vi "CalibrationOAM.vi"() -> ()   [LabVIEW 2015]
uses:
  <vilib>/Utility/file.llb/Write Delimited Spreadsheet (DBL).vi
panel:
  in  "Dimensions":i32=21
  in  "Steps":enum32{"One Step", "Two Step"}(radio)
  out "SLM  B":picture
  out "SLM A":picture
  out "Calibration Curve":dbl[](array[numeric])=[1.04866638e-09, 2.36400149e-10, 3.28397032e-10, 3.4456285e-11, 1.42615789e-11, 6.36260558e-11, 1.65061454e-11, 1.20186092e-11, 3.22117194e-11, 4.34313557e-11, 1.69085523e-10, -3.68856204e-12, 5.28650778e-12, -1.44559289e-12, 7.52947704e-12, 3.04194213e-12, 9.77404269e-12, 3.04194213e-12, 7.52947704e-12, 7.98972867e-13, 3.04194213e-12]
  out "Measured Power":dbl=1.53557755e-09
  out "Generated OAM Progress":u8(slide)=100 scale=0.0..100.0
  out "Current Measured OAM":i32=10
  in  "Measured OAM":i32[](array[numeric])=[-10, -9, -8, -7, -6, -5, -4, -3, -2, -1, 0, 1, 2, 3, 4, 5, 6, 7, 8, 9, 10]
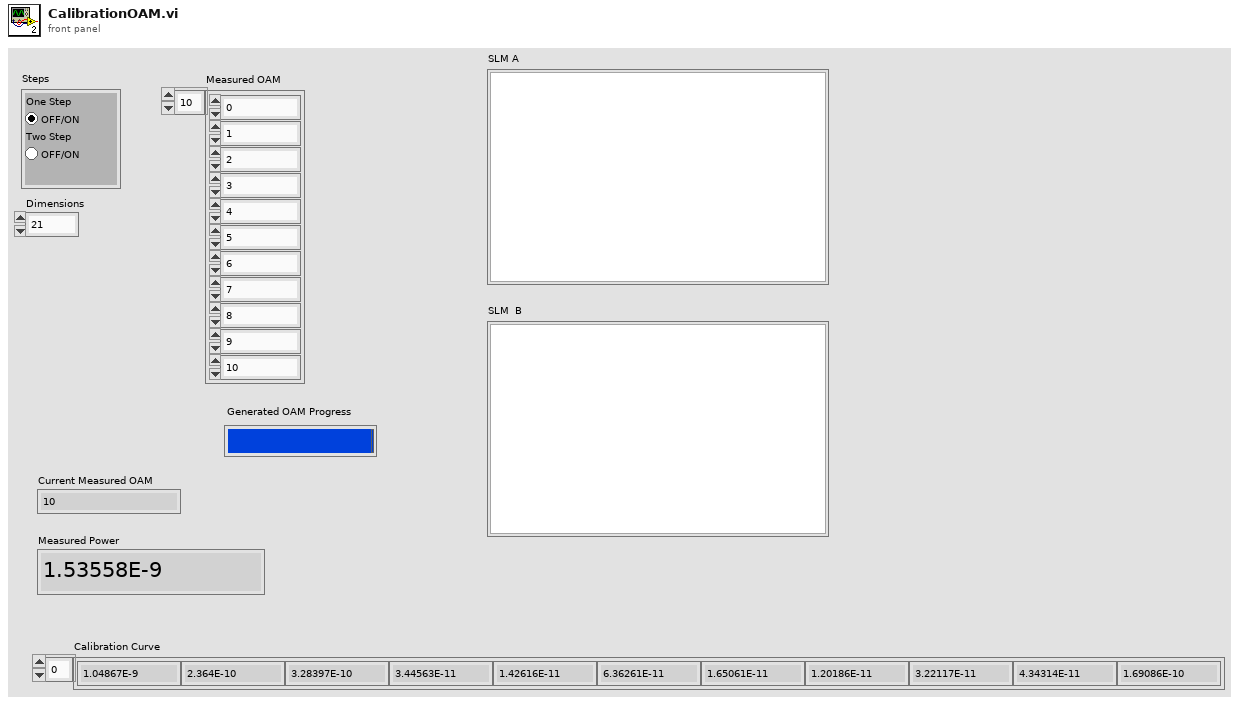
[diagram p1: front panel]
types:
  T1 = cluster{"type":enum16{"Azimuth Mode", "LG mode", "HG mode"}, i32, i32, dbl, dbl}
  T2 = cluster{"type":enum16{"Azimuth Mode", "LG mode", "HG mode"}, "Numeric":i32, i32, dbl, dbl}
  T3 = cluster{"type":enum16{"Azimuth Mode", "LG mode", "HG mode"}, "Numeric":i32, i32, dbl, dbl}[]
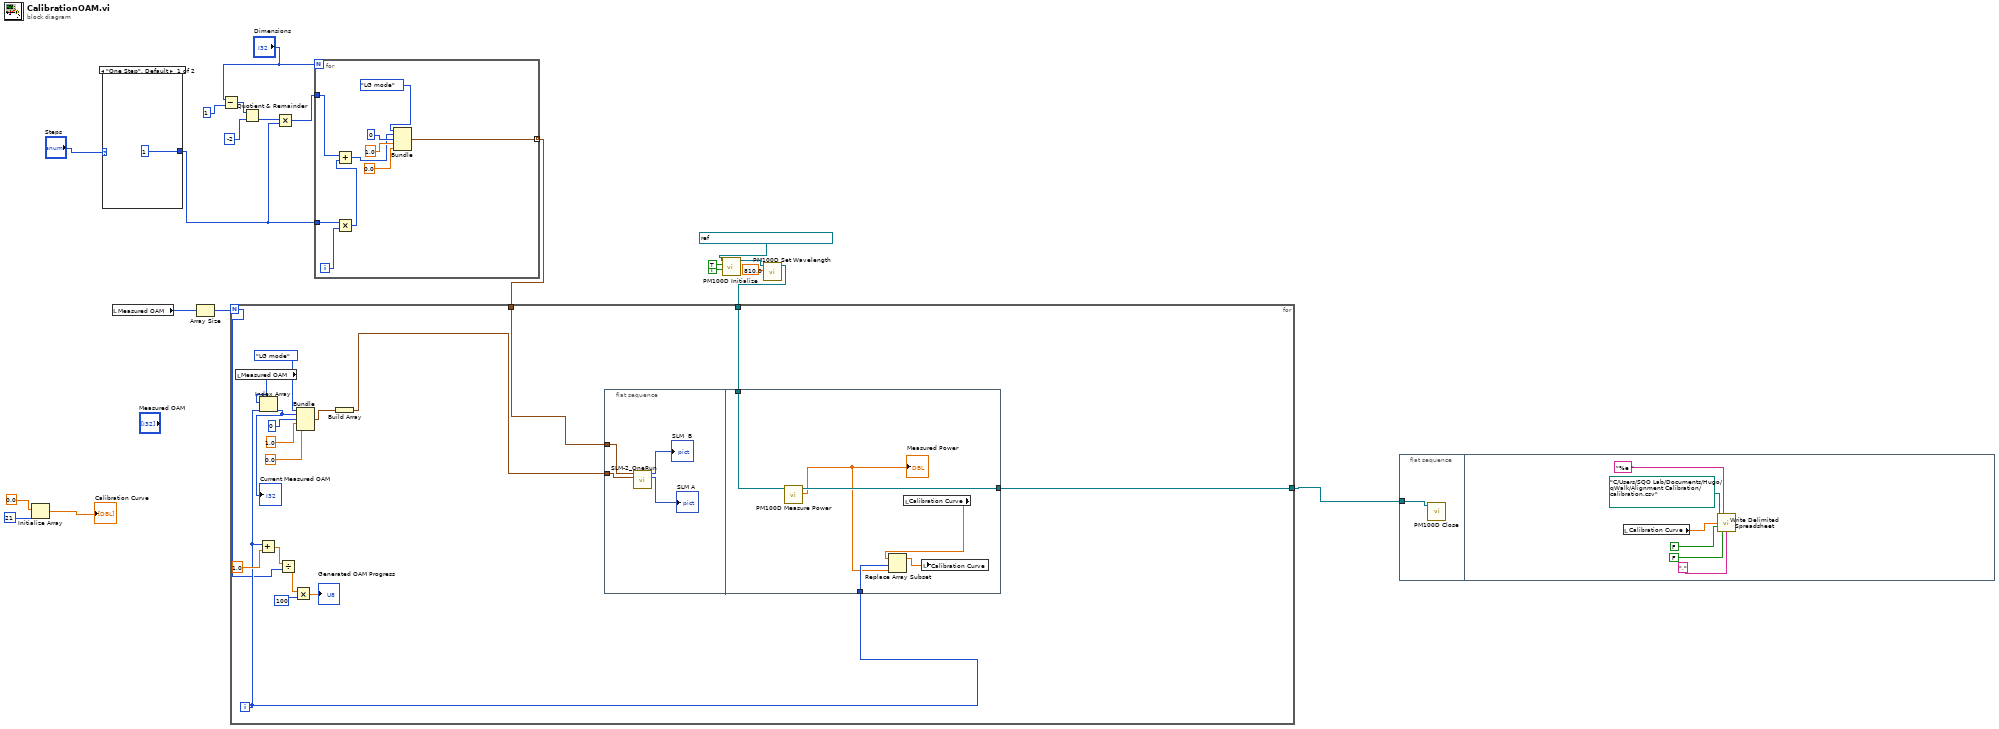
[diagram p0: block diagram]
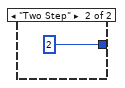
[diagram p2: hidden frame]
diagram:
  n1 = Initialize Array(0.0 ("element"), 21 ("dimension size")) -> (→"Calibration Curve":dbl[])
  n2 = case shown="\"One Step\", Default" "Steps" {
    tunnel: [1 2] -> w2
    frame "One Step", Default {
    }
    frame "Two Step" {
    }
  }
  n3 = local read "Measured OAM"() -> (w21:i32[])
  n4 = Array Size(array=w21) -> (size(s)=w20:i32)
  n5 = Subtract(x="Dimensions", y=1) -> (x-y=w5:i32)
  n6 = Quotient & Remainder(x=w5, y=-2) -> (floor(x/y)=w3:i32)  [unwired: 1 out]
  n7 = Multiply(x=w3, y=w2) -> (x*y=w1:i32)
  n8 = for {
    N: "Dimensions" -> [_]
    tunnel: [w29] -> w4 mode=indexing
    tunnel: w2 -> [w27]
    tunnel: w1 -> [w26]
    i -> [w28]
    n9 = Multiply(x=w27, y=w28) -> (x*y=w25:i32)
    n10 = Add(x=w26, y=w25) -> (x+y=w24:i32)
    n11 = Bundle("type"=enum16{"Azimuth Mode", "LG mode", "HG mode"}."LG mode", w24, 0, 1.0, 0.0) -> (w29:T1)  [unwired: 1 in]
  }
  n12 = call <instrlib>:"PM100D Initialize.vi"("Reset Device (Reset Device)"=TRUE, "ID Query (Do Query)"=TRUE, "resource name"=refnum<visa-resource-name> "USB0::0x1313::0x8078::P0014115::INSTR") -> ("instrument handle out"=w18:refnum<visa-resource-name>)  [unwired: 7 in, 1 out]
  n13 = call <instrlib>:"PM100D Set Wavelength.vi"("Wavelength (0.0)"=810.0, "instrument handle"=w18) -> ("instrument handle out"=w14:refnum<visa-resource-name>)  [unwired: 8 in, 1 out]
  n14 = for {
    N: w20 -> [w36]
    tunnel: w14 -> [w41]
    tunnel: [w40] -> w10
    tunnel: w4 -> [w34]
    i -> [w38]
    n15 = local read "Measured OAM"() -> (w51:i32[])
    n16 = Add(x=w38, y=1.0) -> (x+y=w37:dbl)
    n17 = Index Array(array=w51, index=w38) -> (element=w46:i32)
    "Current Measured OAM" <- w46
    n18 = Divide(x=w37, y=w36) -> (x/y=w35:dbl)
    n19 = Multiply(x=w35, y=100) -> (x*y=→"Generated OAM Progress":dbl)
    n20 = Bundle("type"=enum16{"Azimuth Mode", "LG mode", "HG mode"}."LG mode", "Numeric"=w46, 0, 1.0, 0.0) -> (w43:T2)  [unwired: 1 in]
    n21 = Build Array(w43) -> (w42:T3)
    n22 = flat-sequence {
      tunnel: w34 -> [w52]
      tunnel: w42 -> [w55]
      tunnel: w38 -> [w59]
      tunnel: w41 -> [w58]
      tunnel: [w57] -> w40
      frame #0 {
        n23 = call "SLM-2_OneRun.vi"("Modes B - SLM 2"=w55, "Modes - UV"=w52) -> ("SLM"=→"SLM A":picture, "SLM  B"=→"SLM  B":picture)  [unwired: 8 in]
      }
      frame #1 {
        n24 = call <instrlib>:"PM100D Measure Power.vi"("instrument handle"=w58) -> ("Power"=w56:dbl, "instrument handle out"=w57:refnum<visa-resource-name>)  [unwired: 8 in, 1 out]
        "Measured Power" <- w56
        n25 = local read "Calibration Curve"() -> (w61:dbl[])
        n26 = Replace Array Subset(array=w61, new element=w56, index=w59) -> (w60:dbl[])
        n27 = local write "Calibration Curve"(w60) -> ()
      }
    }
  }
  n28 = flat-sequence {
    tunnel: w10 -> [w62]
    frame #0 {
      n29 = call <instrlib>:"PM100D Close.vi"("instrument handle"=w62) -> ()  [unwired: 10 in, 1 out]
    }
    frame #1 {
      n30 = local read "Calibration Curve"() -> (w63:dbl[])
      n31 = call-poly <vilib>:"Write Delimited Spreadsheet.vi"("file path (dialog if empty)"=path "C:/Users/SQO Lab/Documents/Hugo/qWalk/Alignment Calibration/calibration.csv", "format (%.3f)"="%e ", "1D data"=w63, "append to file? (F)"=FALSE, "transpose? (F)"=FALSE, "delimiter (\\t)"=",") -> ()  [unwired: 8 in, 2 out]
    }
  }
